vi "init classes.vi"(8 "error in (no error)":errorcluster, 9 "Param Referense":T1, 10 "Data Reference":T2, 11 "Status Reference":T3) -> (0 "error out":errorcluster, 3 "classes":refnum<class "MB_TCP.lvclass">[](array[class]))   [LabVIEW 2021, in "MB_TCP.lvclass"]
uses:
  MB_TCP.lvclass
  ICPCON ET-7018/ICPCON ET-7018.lvclass
  ICPCON ET-7016/ICPCON ET-7016.lvclass
  Master CR/Devices/ET7000/ICPCON ET-7051/ICPCON ET-7051.lvclass
  Master CR/Devices/ET7000/ICPCON ET-7017/ICPCON ET-7017.lvclass
  Master CR/Devices/ET7000/ICPCON ET-7018i/ICPCON ET-7018i.lvclass
  ICPCON ET-7024i/ICPCON ET-7024i.lvclass
  ZERO/ZERO.lvclass
  NS300/NS300.lvclass
  ICPCON ET-7042i/ICPCON ET-7042i.lvclass
  Master CR/Devices/ET7000/TEST/TEST.lvclass
  LIR-919D/LIR-919D.lvclass
  Master CR/Devices/ET7000/ICPCON ET-7016i/ICPCON ET-7016i.lvclass
  Master CR/Devices/ET7000/ICPCON ET-7024/ICPCON ET-7024.lvclass
  Master CR/Devices/SMSD/SMSD-AI/SMSD-AI.lvclass
  Master CR/Devices/SMSD/SMSD-DI/SMSD-DI.lvclass
  Master CR/Devices/ET7000/ICPCON ET-7028/ICPCON ET-7028.lvclass
  Master CR/Devices/OHAUS_Navigator/OHAUS_Navigator.lvclass
  tGw-TEST1/tGw-TEST1.lvclass
  Master CR/Devices/ET7000/ICPCON ET-7042/ICPCON ET-7042.lvclass
  ICPCON ET-7024ao/ICPCON ET-7024ao.lvclass
  Serial/OHAUS_Navigator_232/OHAUS_Navigator_232.lvclass
  D:/my_projects/projects/Algorithms/Labview/21/WebSockets/Source/Unit Tests/Test WebSockets Server/MB_TCP2/MB_TCP.lvclass
  D:/my_projects/projects/Algorithms/Labview/21/WebSockets/Source/Unit Tests/Test WebSockets Server/MB_TCP2/ZERO/ZERO.lvclass
  D:/my_projects/projects/Algorithms/Labview/21/WebSockets/Source/Unit Tests/Test WebSockets Server/MB_TCP2/ICPCON ET-7016/ICPCON ET-7016.lvclass
  D:/my_projects/projects/Algorithms/Labview/21/WebSockets/Source/Unit Tests/Test WebSockets Server/NI_modbus_upd/TCP/TCP.lvclass
  D:/my_projects/projects/Algorithms/Labview/21/Master CR/Devices/ET7000/ICPCON ET-7016i/ICPCON ET-7016i.lvclass
  D:/my_projects/projects/Algorithms/Labview/21/Master CR/Devices/ET7000/ICPCON ET-7017/ICPCON ET-7017.lvclass
  D:/my_projects/projects/Algorithms/Labview/21/WebSockets/Source/Unit Tests/Test WebSockets Server/MB_TCP2/ICPCON ET-7018/ICPCON ET-7018.lvclass
  D:/my_projects/projects/Algorithms/Labview/21/Master CR/Devices/ET7000/ICPCON ET-7018i/ICPCON ET-7018i.lvclass
  D:/my_projects/projects/Algorithms/Labview/21/Master CR/Devices/ET7000/ICPCON ET-7024/ICPCON ET-7024.lvclass
  D:/my_projects/projects/Algorithms/Labview/21/WebSockets/Source/Unit Tests/Test WebSockets Server/MB_TCP2/ICPCON ET-7024i/ICPCON ET-7024i.lvclass
  D:/my_projects/projects/Algorithms/Labview/21/WebSockets/Source/Unit Tests/Test WebSockets Server/MB_TCP2/ICPCON ET-7024ao/ICPCON ET-7024ao.lvclass
  D:/my_projects/projects/Algorithms/Labview/21/Master CR/Devices/ET7000/ICPCON ET-7028/ICPCON ET-7028.lvclass
  D:/my_projects/projects/Algorithms/Labview/21/WebSockets/Source/Unit Tests/Test WebSockets Server/MB_TCP2/ICPCON ET-7042i/ICPCON ET-7042i.lvclass
  D:/my_projects/projects/Algorithms/Labview/21/Master CR/Devices/ET7000/ICPCON ET-7042/ICPCON ET-7042.lvclass
  D:/my_projects/projects/Algorithms/Labview/21/Master CR/Devices/ET7000/ICPCON ET-7051/ICPCON ET-7051.lvclass
  D:/my_projects/projects/Algorithms/Labview/21/WebSockets/Source/Unit Tests/Test WebSockets Server/MB_TCP2/NS300/NS300.lvclass
  D:/my_projects/projects/Algorithms/Labview/21/Master CR/Devices/ET7000/TEST/TEST.lvclass
  D:/my_projects/projects/Algorithms/Labview/21/WebSockets/Source/Unit Tests/Test WebSockets Server/MB_TCP2/LIR-919D/LIR-919D.lvclass
  D:/my_projects/projects/Algorithms/Labview/21/Master CR/Devices/SMSD/SMSD.lvclass
  D:/my_projects/projects/Algorithms/Labview/21/Master CR/Master CR.lvclass
  D:/my_projects/projects/Algorithms/Labview/21/Master CR/Devices/SMSD/SMSD-AI/SMSD-AI.lvclass
  D:/my_projects/projects/Algorithms/Labview/21/Master CR/Devices/SMSD/SMSD-DI/SMSD-DI.lvclass
  D:/my_projects/projects/Algorithms/Labview/21/WebSockets/Source/Unit Tests/Test WebSockets Server/MB_TCP2/tGw-TEST1/tGw-TEST1.lvclass
  D:/my_projects/projects/Algorithms/Labview/21/Serial/OHAUS_Navigator_232/OHAUS_Navigator_232.lvclass
  Eth Status/Ctl/Status.ctl
  Eth Status/Eth Status.lvlib
  ICPCON Registers/Ctl/ICPCON Data.ctl
  ICPCON Registers/ICPCON Registers.lvlib
  ICPCON Param/ICPCON Param.ctl
  ICPCON Param/ICPCON_Param.lvlib
  MB_TCP_State.ctl
  ICPCON Param/Eth timeouts.ctl
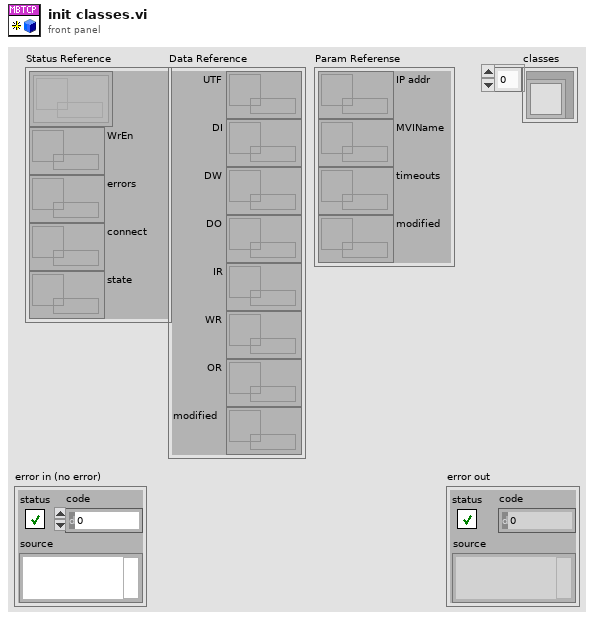
[diagram p1: front panel]
types:
  T1 = typedef "ICPCON_Param.lvlib/ICPCON Param.ctl" = cluster{"IP addr":refnum<data-value>, "MVIName":refnum<data-value>, "timeouts":refnum<data-value>, "modified":refnum<data-value>}
  T2 = typedef "ICPCON Registers.lvlib/ICPCON Data.ctl" = cluster{"UTF":refnum<data-value>, "DI":refnum<data-value>, "DW":refnum<data-value>, "DO":refnum<data-value>, "IR":refnum<data-value>, "WR":refnum<data-value>, "OR":refnum<data-value>, "modified":refnum<data-value>}
  T3 = typedef "Eth Status.lvlib/Status.ctl" = cluster{"Set_states":refnum<queue>[], "WrEn":refnum<data-value>, "errors":refnum<data-value>, "connect":refnum<data-value>, "state":refnum<data-value>}
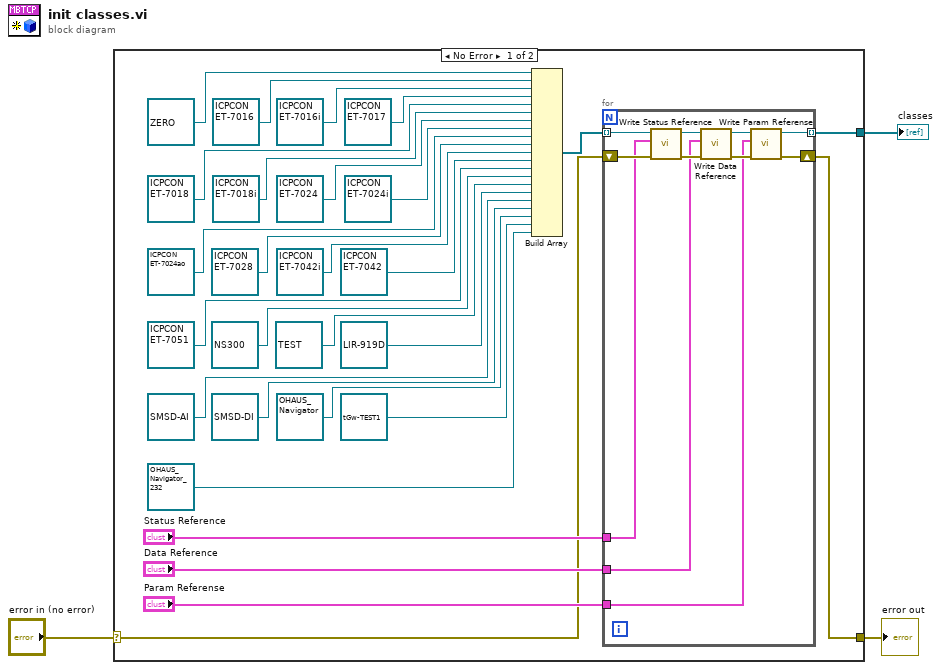
[diagram p0: block diagram]
diagram:
  n1 = case shown="No Error" "error in (no error)" {
    selector: "error in (no error)" -> [w27 w43]
    tunnel: [w26 w43] -> w2
    tunnel: [w28 _] -> w1
    frame No Error {
      n2 = Build Array(refnum<class "ZERO.lvclass"> refnum ("ZERO.lvclass"), refnum<class "ICPCON ET-7016.lvclass"> refnum ("ICPCON ET-7016.lvclass"), refnum<class "ICPCON ET-7016i.lvclass"> refnum ("ICPCON ET-7016i.lvclass"), refnum<class "ICPCON ET-7017.lvclass"> refnum ("ICPCON ET-7017.lvclass"), refnum<class "ICPCON ET-7018.lvclass"> refnum ("ICPCON ET-7018 in"), refnum<class "ICPCON ET-7018i.lvclass"> refnum ("ICPCON ET-7018i.lvclass"), refnum<class "ICPCON ET-7024.lvclass"> refnum ("ICPCON ET-7024.lvclass"), refnum<class "ICPCON ET-7024i.lvclass"> refnum ("ICPCON ET-7024i.lvclass"), refnum<class "ICPCON ET-7024ao.lvclass"> refnum ("ICPCON ET-7024ao.lvclass"), refnum<class "ICPCON ET-7028.lvclass"> refnum ("ICPCON ET-7028.lvclass"), refnum<class "ICPCON ET-7042i.lvclass"> refnum ("ICPCON ET-7042i.lvclass"), refnum<class "ICPCON ET-7042.lvclass"> refnum ("ICPCON ET-7042.lvclass"), refnum<class "ICPCON ET-7051.lvclass"> refnum ("ICPCON ET-7051.lvclass"), refnum<class "NS300.lvclass"> refnum ("NS300.lvclass"), refnum<class "TEST.lvclass"> refnum ("TEST.lvclass"), refnum<class "LIR-919D.lvclass"> refnum ("LIR-919D.lvclass"), refnum<class "SMSD-AI.lvclass"> refnum ("SMSD-AI.lvclass"), refnum<class "SMSD-DI.lvclass"> refnum ("SMSD-DI.lvclass"), refnum<class "OHAUS_Navigator.lvclass"> refnum ("OHAUS_Navigator.lvclass"), refnum<class "tGw-TEST1.lvclass"> refnum ("tGw-TEST1.lvclass"), refnum<class "OHAUS_Navigator_232.lvclass"> refnum ("OHAUS_Navigator_232.lvclass")) -> (w11:refnum<class>[])
      n3 = for {
        shift-right: [w36] -> w26
        shift-left: w27 -> [w37]
        tunnel: w11 -> [w38] mode=indexing
        tunnel: "Status Reference" -> [w35]
        tunnel: "Data Reference" -> [w34]
        tunnel: "Param Referense" -> [w33]
        tunnel: [w32] -> w28 mode=indexing
        n4 = call "Write Status Reference.vi"("error in (no error)"=w37, "Status"=w35, "MB_TCP in"=w38) -> ("error out"=w40:errorcluster, "MB_TCP out"=w39:refnum<class "MB_TCP.lvclass">)  [unwired: 7 in]
        n5 = call "Write Data Reference.vi"("error in (no error)"=w40, "Data"=w34, "MB_TCP in"=w39) -> ("error out"=w42:errorcluster, "MB_TCP out"=w41:refnum<class "MB_TCP.lvclass">)  [unwired: 7 in]
        n6 = call "Write Param Referense.vi"("error in (no error)"=w42, "Param Referense"=w33, "MB_TCP in"=w41) -> ("error out"=w36:errorcluster, "MB_TCP out"=w32:refnum<class "MB_TCP.lvclass">)  [unwired: 7 in]
      }
    }
    frame Error {
    }
  }
  "error out" <- w2
  "classes" <- w1
